vi "Initialize Session.vi"(6 "initialize and close session behavior":T1, 8 "error in":errorcluster, 9 "Option String":string, 10 "Reset":bool, 11 "session reservation in":refnum<class "Session Reservation.lvclass">) -> (0 "error out":errorcluster, 1 "channel list":string, 2 "session":refnum<k15>, 3 "session reservation out":refnum<class "Session Reservation.lvclass">)   [LabVIEW 2020, in "IVI Scope Instrument.lvlib"]
uses:
  IVI Scope Instrument.lvlib
  <vilib>/MeasurementLink/MeasurementLink Session Management V1/Session Reservation/Initialize and Close Session Behavior.ctl
  <vilib>/MeasurementLink/MeasurementLink Session Management V1/Session Reservation/Session Reservation.lvclass
  d6b68087-02be-4672-9a92-db6824c7b8ca.vi
  Session Factory/Session Factory.lvclass
  C:/Program Files/National Instruments/LabVIEW 2020/vi.lib/MeasurementLink/MeasurementLink Instrument/ISession Factory/ISession Factory.lvclass
  <vilib>/MeasurementLink/MeasurementLink Session Management V1/Session Reservation/Initialize Sessions with Retry.vi
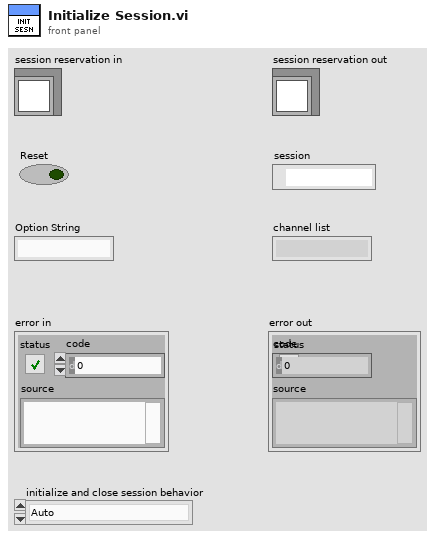
[diagram p1: front panel]
types:
  T1 = typedef "MeasurementLink Session Management V1.lvlib/Session Reservation.lvclass/Initialize and Close Session Behavior.ctl" = enum16{"Auto", "Initialize and Close", "Attach and Detach", "Initialize and Detach", "Attach and Close"}
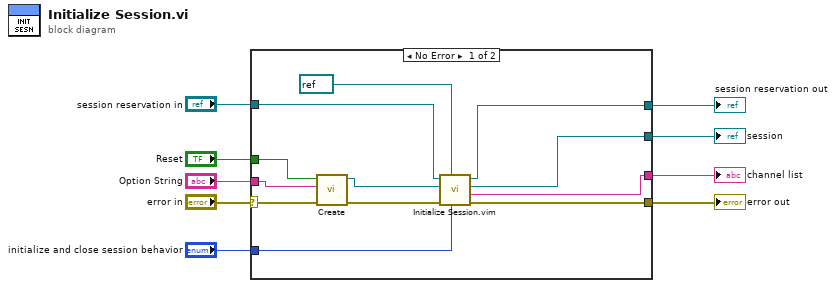
[diagram p0: block diagram]
diagram:
  n1 = case shown="No Error" "error in" {
    selector: "error in" -> [w16 w23]
    tunnel: "initialize and close session behavior" -> [w21 _]
    tunnel: [w20 w23] -> w7
    tunnel: "Reset" -> [w18 _]
    tunnel: "Option String" -> [w17 _]
    tunnel: "session reservation in" -> [w13 w22]
    tunnel: [w12 w22] -> w3
    tunnel: [w11 _] -> w2
    tunnel: [w10 _] -> w1
    frame No Error {
      n2 = call "Create.vi"("error in"=w16, "Option String"=w17, "Reset"=w18) -> ("error out"=w15:errorcluster, "Session Factory Out"=w14:refnum<class "Session Factory.lvclass">)  [unwired: 7 in]
      n3 = call "Initialize Session.vim"("initialize and close session behavior"=w21, "session type"=refnum<k15> refnum ("instrument handle"), "error in"=w15, "session factory"=w14, "session reservation in"=w13) -> ("error out"=w20:errorcluster, "channel list"=w10:string, "session"=w11:refnum<k15>, "session reservation out"=w12:refnum<class "Session Reservation.lvclass">)  [unwired: 3 in]
    }
    frame Error {
    }
  }
  "error out" <- w7
  "session reservation out" <- w3
  "session" <- w2
  "channel list" <- w1
